vi "Clean Up MeasurementLink Session for Init Error.vi"(8 "error in":errorcluster, 9 "initialize and close session behavior":T1, 10 "session in":variant, 11 "instrument in":refnum<class "IInstrument.lvclass">) -> (0 "error out":errorcluster)   [LabVIEW 2020, in "MeasurementLink Instrument.lvlib" / "IInstrument.lvclass"]
doc: "Closes the local session in the event that an error occurred while creating a set of sessions. If the session represents a remote session, <b>initialize and close session behavior</b> indicates whether the remote session was created or attached to when initializing the local session. The default implementation sends \"Create and Close\" or \"Attach and Detach\" respectively to the \"Close MeasurementLink Session\" VI."
uses:
  IInstrument.lvclass
  Initialize and Close Session Behavior.ctl
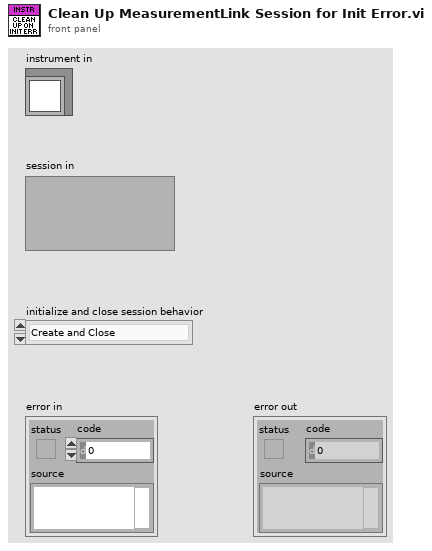
[diagram p1: front panel]
types:
  T1 = typedef "MeasurementLink Instrument.lvlib/IInstrument.lvclass/Initialize and Close Session Behavior.ctl" = enum16{"Create and Close", "Attach and Detach", "Create and Detach", "Attach and Close"}
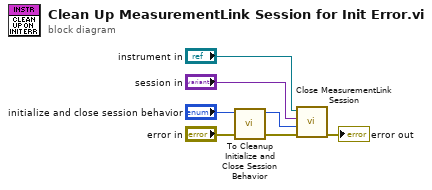
[diagram p0: block diagram]
diagram:
  n1 = call "To Cleanup Initialize and Close Session Behavior.vi"("initialize and close session behavior"="initialize and close session behavior") -> ("cleanup initialize and close session behavior"=w1:T1)  [unwired: 10 in]
  n2 = call-dynamic "Close MeasurementLink Session.vi"("error in (no error)"="error in", "initialize and close session behavior"=w1, "session in"="session in", "instrument in"="instrument in") -> ("error out"=→"error out":errorcluster)  [unwired: 7 in]
